vi "True.vi"() -> (1 "Booléen":bool)   [LabVIEW 2012]
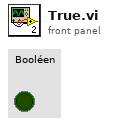
[diagram p1: front panel]
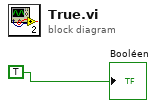
[diagram p0: block diagram]
diagram:
  "Booléen" <- TRUE
